vi "ASCI TO HEX.vi"(11 "ASCII":string) -> (2 "数字":u32, 3 "HEX":string)   [LabVIEW 2015, in "PLC.lvlib"]
uses:
  PLC.lvlib
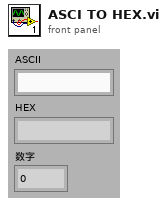
[diagram p1: front panel]
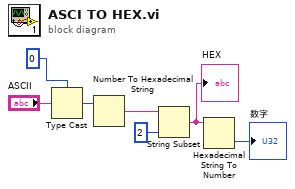
[diagram p0: block diagram]
diagram:
  n1 = Type Cast(type=0, x="ASCII") -> (*(type *) &x=w5:i32)
  n2 = Number To Hexadecimal String(2:w5) -> (0:w2:string)  [unwired: 1 out]
  n3 = String Subset(string=w2, length (rest)=2 ("长度（剩余）")) -> (substring=w1:string)  [unwired: 1 out]
  "HEX" <- w1
  n4 = Hexadecimal String To Number(string=w1) -> (number=→"数字":u32)  [unwired: 3 out]
